vi "Manual Override Speed Calculation.vi"(11 "Input":dbl) -> (2 "Output":dbl)   [LabVIEW 2011]
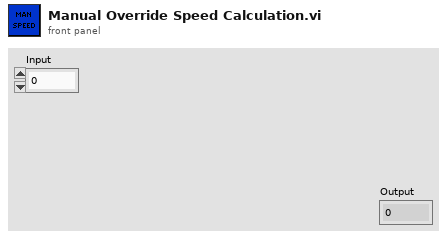
[diagram p1: front panel]
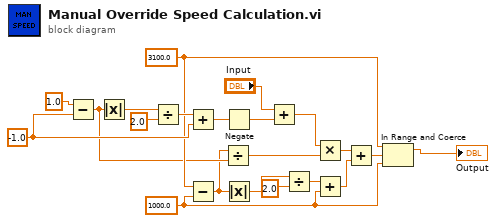
[diagram p0: block diagram]
diagram:
  w6 = 1000.0 ("Output Min")
  w5 = 3100.0 ("Output Max")
  w15 = -1.0 ("Input Min")
  n1 = Subtract(x=1.0 ("Input Max"), y=w15) -> (x-y=w3:dbl)
  n2 = Absolute Value(x=w3) -> (abs(x)=w21:dbl)
  n3 = Divide(x=w21, y=2.0 ("x")) -> (x/y=w16:dbl)
  n4 = Add(x=w16, y=w15) -> (x+y=w14:dbl)
  n5 = Subtract(x=w5, y=w6) -> (x-y=w2:dbl)
  n6 = Divide(x=w2, y=w3) -> (x/y=w10:dbl)
  n7 = Negate(x=w14) -> (-x=w18:dbl)
  n8 = Absolute Value(x=w2) -> (abs(x)=w20:dbl)
  n9 = Add(x="Input", y=w18) -> (x+y=w11:dbl)
  n10 = Divide(x=w20, y=2.0 ("x")) -> (x/y=w12:dbl)
  n11 = Multiply(x=w11, y=w10) -> (x*y=w9:dbl)
  n12 = Add(x=w12, y=w6) -> (x+y=w8:dbl)
  n13 = Add(x=w9, y=w8) -> (x+y=w7:dbl)
  n14 = In Range and Coerce(upper limit=w5, x=w7, lower limit=w6) -> (coerced(x)=→"Output":dbl)  [unwired: 1 out]
